vi "摆角范围判断（起摆）-子.vi"(1 "摆臂角度":dbl) -> (0 "判断摆角是否在（10,165）或（-165，-10）范围内——起摆":bool)   [LabVIEW 2015]
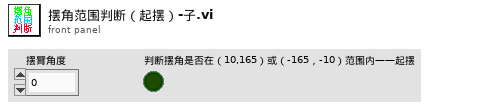
[diagram p1: front panel]
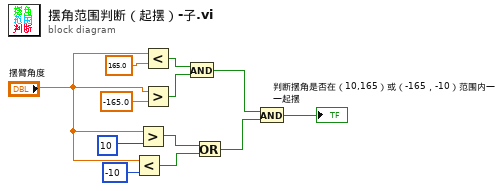
[diagram p0: block diagram]
diagram:
  n1 = Less?(x="摆臂角度", y=-10) -> (x < y?=w7:bool)
  n2 = Greater?(x="摆臂角度", y=10) -> (0:w9:bool)
  n3 = Less?(x="摆臂角度", y=165.0) -> (x < y?=w11:bool)
  n4 = Greater?(x="摆臂角度", y=-165.0) -> (0:w3:bool)
  n5 = And(x=w11, y=w3) -> (x .and. y?=w5:bool)
  n6 = Or(x=w9, y=w7) -> (x .or. y?=w6:bool)
  n7 = And(x=w5, y=w6) -> (x .and. y?=→"判断摆角是否在（10,165）或（-165，-10）范围内——起摆":bool)
